vi "Initialize.vi"(8 "error in (no error)":errorcluster, 10 "Stage Comms":T1={"CommsProtocol.lvclass"=refnum, "CommsProtocol.lvclass 2"=refnum, "CommsProtocol.lvclass 3"=refnum, "XYZ Control Config"=enum."XYZ", "Translation Stage Description"=""}, 11 "XYZ Stage Control in":refnum<class "XYZ Stage Control.lvclass">) -> (0 "error out":errorcluster, 3 "XYZ Stage Control out":refnum<class "XYZ Stage Control.lvclass">)   [LabVIEW 2020, in "TranslationStageClassStructure.lvlib" / "XYZ Stage Control.lvclass"]
uses:
  XYZ Stage Control.lvclass
  typedefs/TranslationStageControlInfo.ctl
  Generic Comms/CommsProtocol/CommsProtocol.lvclass
  typedefs/XYZControlConfig.ctl
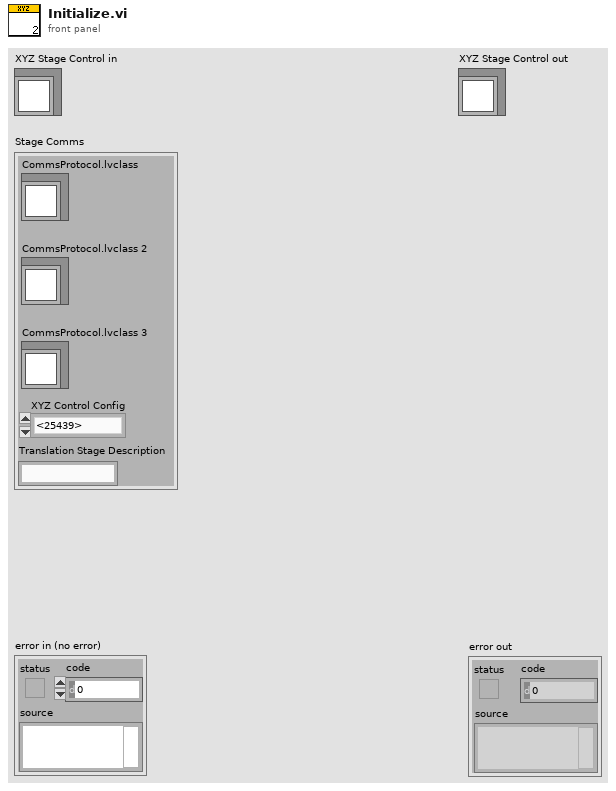
[diagram p1: front panel]
types:
  T1 = typedef "TranslationStageControlInfo.ctl" = cluster{"CommsProtocol.lvclass":refnum<class "CommsProtocol.lvclass">, "CommsProtocol.lvclass 2":refnum<class "CommsProtocol.lvclass">, "CommsProtocol.lvclass 3":refnum<class "CommsProtocol.lvclass">, "XYZ Control Config":T2, "Translation Stage Description":string}
  T2 = typedef "XYZControlConfig.ctl" = enum16{"None", "XYZ", "XY-Z", "X-Y-Z", "Z"}
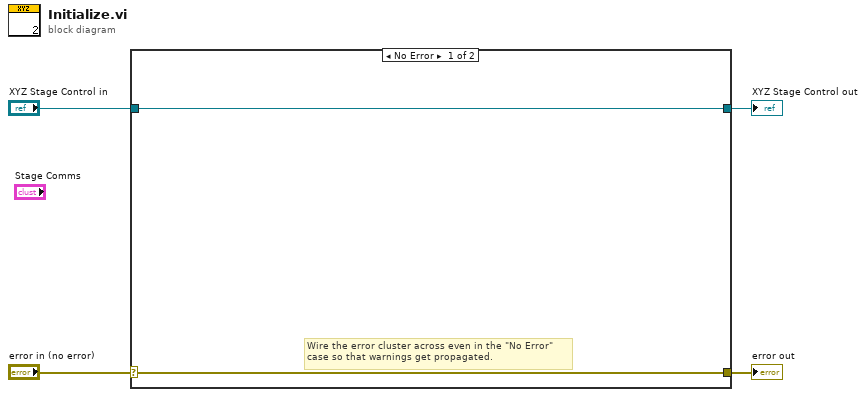
[diagram p0: block diagram]
diagram:
  n1 = case shown="No Error" "error in (no error)" {
    selector: "error in (no error)" -> [w5 w8]
    tunnel: [w5 w8] -> w3
    tunnel: [w6 w7] -> w1
    tunnel: "XYZ Stage Control in" -> [w6 w7]
    frame No Error {
      # "Wire the error cluster across even in the \"No Error\"\ncase so that warnings get propagated."
    }
    frame Error {
    }
  }
  "error out" <- w3
  "XYZ Stage Control out" <- w1
